vi "Set Camera Configuration.vi"(8 "error in (no error)":errorcluster, 10 "Configuration":T1, 11 "NI Vision Camera in":refnum<class "NI Vision Camera.lvclass">) -> (0 "error out":errorcluster, 3 "NI Vision Camera out":refnum<class "NI Vision Camera.lvclass">)   [LabVIEW 2014, in "NI Vision Camera.lvclass"]
uses:
  NI Vision Camera.lvclass
  NI Vision Camera Device/Configuration.ctl
  NI Vision Camera.lvclass/NI Vision Camera.ctl
  NI Vision Camera Device/NI Vision Camera Device.lvclass
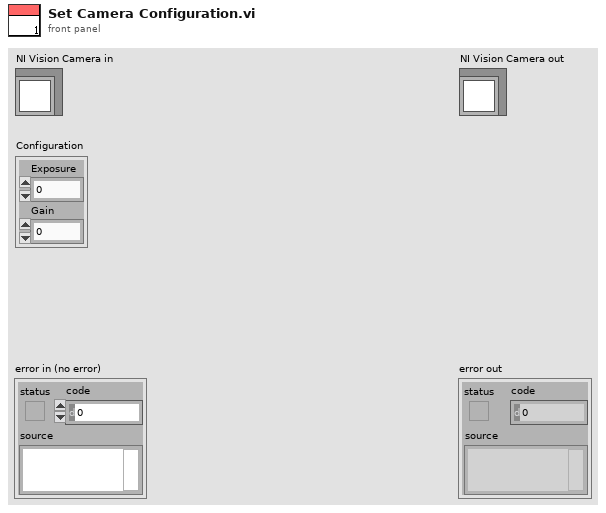
[diagram p1: front panel]
types:
  T1 = typedef "NI Vision Camera Device.lvclass/Configuration.ctl" = cluster{"Exposure":dbl, "Gain":dbl}
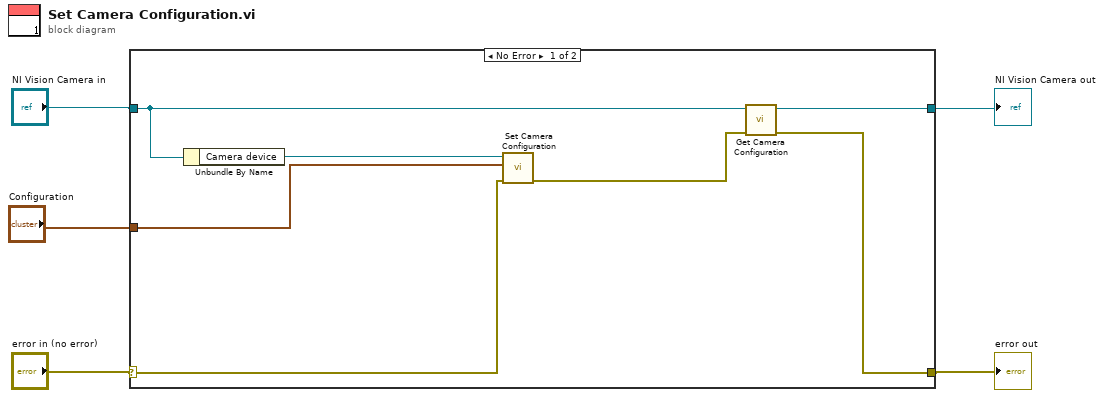
[diagram p0: block diagram]
diagram:
  n1 = case shown="No Error" "error in (no error)" {
    selector: "error in (no error)" -> [w8 w14]
    tunnel: [w10 w14] -> w4
    tunnel: [w11 w13] -> w5
    tunnel: "NI Vision Camera in" -> [w12 w13]
    tunnel: "Configuration" -> [w7 _]
    frame No Error {
      n2 = Unbundle By Name(w12) -> ("Camera device"=w9:refnum<class "NI Vision Camera Device.lvclass">)
      n3 = call "Set Camera Configuration.vi"("error in (no error)"=w8, "Configuration"=w7, "NI Vision Camera in"=w9) -> ("error out"=w6:errorcluster)  [unwired: 7 in, 1 out]
      n4 = call "Get Camera Configuration.vi"("error in (no error)"=w6, "NI Vision Camera in"=w12) -> ("error out"=w10:errorcluster, "NI Vision Camera out"=w11:refnum<class "NI Vision Camera.lvclass">)  [unwired: 7 in, 1 out]
    }
    frame Error {
    }
  }
  "error out" <- w4
  "NI Vision Camera out" <- w5
